vi "ExperimentCode_Serial.vi"() -> ()   [LabVIEW 2017]
uses:
  <vilib>/Analysis/baseanly.llb/Mean (DBL).vi
  <vilib>/Instr/_visa.llb/VISA Configure Serial Port (Instr).vi
  <vilib>/express/express shared/transition.llb/Dynamic To Waveform Array.vi
  <vilib>/express/express signal manip/GetorSetDDTAttributes/Set DDT Attributes/SetT0.vi
  <vilib>/express/express shared/transition.llb/Waveform Array To Dynamic.vi
  <vilib>/express/express signal manip/GetorSetDDTAttributes/Set DDT Attributes/Set DDT Properties.xnode
  <vilib>/Analysis/NI_AALBase.lvlib
panel:
  in  "Tab Control":enum32{"Setup ", "Experiment Controls", "Debug"}(tab)=enum."Experiment Controls"
  in  "Max Torque":dbl=21.3
  in  "Servo 1 Zero Offset":dbl=-9.0
  in  "Servo 2 Zero Offset":dbl=10.0
  in  "Servo 3 Zero Offset":dbl=-9.0
  in  "Servo 4 Zero Offset":dbl
  in  "Servo 5 Zero Offset":dbl
  in  "Servo 5 Torque Intercept":dbl
  in  "Servo 5 Torque Slope":dbl=1.0
  in  "Servo 5 Position Intercept":dbl
  in  "Servo 5 Position Slope":dbl=1.0
  in  "Servo 4 Torque Intercept":dbl=-72.1928
  in  "Servo 4 Torque Slope":dbl=0.002332
  in  "Servo 4 Position Intercept":dbl=97.9723
  in  "Servo 4 Position Slope":dbl=-0.00488
  in  "Servo 3 Torque Intercept":dbl
  in  "Servo 3 Torque Slope":dbl=1.0
  in  "Servo 3 Position Intercept":dbl
  in  "Servo 3 Position Slope":dbl=1.0
  in  "Servo 2 Torque Intercept":dbl
  in  "Servo 2 Torque Slope":dbl=1.0
  in  "Servo 2 Position Intercept":dbl
  in  "Servo 2 Position Slope":dbl=1.0
  in  "Servo 1 Torque Intercept":dbl
  in  "Servo 1 Torque Slope":dbl=1.0
  in  "Servo 1 Position Intercept":dbl
  in  "Servo 1 Position Slope":dbl=1.0
  in  "Plot Last x Seconds":dbl=100.0
  in  "COM Port":refnum<visa-resource-name>
  in  "Buad Rate":i32(ring)=115200 items=["2400"=2400, "4800"=4800, "9600"=9600, "14400"=14400, "19200"=19200, "28800"=28800, "38400"=38400, "57600"=57600, "115200"=115200]
  in  "Lowest Servo Angle":dbl=-65.0
  in  "Highest Servo Angle":dbl=65.0
  in  "Number of Servos":dbl=3.0
  out "Maximum Torque Exceeded":bool
  in  "Amplitude (deg)":dbl=3.0
  in  "Save":bool
  in  "Stop VI":bool
  in  "Sample Frequency":dbl=100.0 step=50.0
  out "Servo Torque":cluster{" Time Offset":dbl, dbl, dbl[][]}(graph)
  in  "Amplitude (cm)":dbl=2.0
  in  "Length of Segments":dbl=10.0
  in  "Number of Waves":dbl=1.0
  in  "Wave Exponential":dbl=2.0
  in  "Frequency":dbl=1.0
  in  "Wave Form":u16(ring) items=["Sine", "Exponentional Sine", "Second Mode Bending", "Flat Plate"]
  in  "Wind Up Waveform":bool
  in  "Mode 1 Amplitude":dbl=0.1 step=0.1
  in  "Mode 2 Amplitude":dbl=0.2 step=0.1
  in  "Mode 1 Phase":dbl step=0.1
  in  "Mode 2 Phase":dbl=0.8499 step=0.1
  in  "Wind Down Waveform":bool
  in  "Wind Down Time":i32=5
  out "Waveform":cluster{"X Nodes":dbl[], "Y Nodes":dbl[]}[](graph)
  in  "Servo Input":bool
  in  "Send To Waveform to MBE":bool
  in  "Servo 5 Input":dbl
  in  "Servo 4 Input":dbl
  in  "Servo 3 Input":dbl
  in  "Servo 2 Input":dbl
  in  "Servo 1  Input":dbl
  out "Minimum or Maximum Angle Exceeded":bool
  in  "Filename":path=path "test.tdms"
  in  "Comment":string
  out "Calculated Sample Frequency":dbl
  out "Specified Time Delay":dbl
  out "Calculated Time Delay":dbl
  out "Time Elapsed":dbl
  out "Output Angles":dbl[](array[numeric])
  out "Input Angles":dbl[](array[numeric])
  out "Pos5 number":dbl
  out "Pos4 number":dbl
  out "Pos3 number":dbl
  out "Pos2 number":dbl
  out "Pos1 number":dbl
  out "Torq1 number":dbl
  out "Torq2 number":dbl
  out "Torq3 number":dbl
  out "Torq4 number":dbl
  out "Torq5 number":dbl
  out "Servo 1 Position":cluster{" Time Offset":dbl, "mean":dbl, dbl[][]}(graph)
  out "Servo 2 Position":cluster{" Time Offset":dbl, "mean":dbl, dbl[][]}(graph)
  out "Servo 3 Position":cluster{" Time Offset":dbl, "mean":dbl, dbl[][]}(graph)
  out "Servo 4 Position":cluster{" Time Offset":dbl, "mean":dbl, dbl[][]}(graph)
  out "Servo 5 Position":cluster{" Time Offset":dbl, "mean":dbl, dbl[][]}(graph)
  out "Sent to Arduino":string
  out "Bytes at port":cluster{i32, dbl, dbl[]}(graph)
  out "Read Buffer":string
  # "deg"
  # "deg"
  # "deg"
  # "deg"
  # "deg"
  # "Waveform"
  # "Manual"
  # "cm"
  # "Hz"
  # "Off"
  # "On"
  # "rad"
  # "rad"
  # "Off"
  # "On"
  # "Hz"
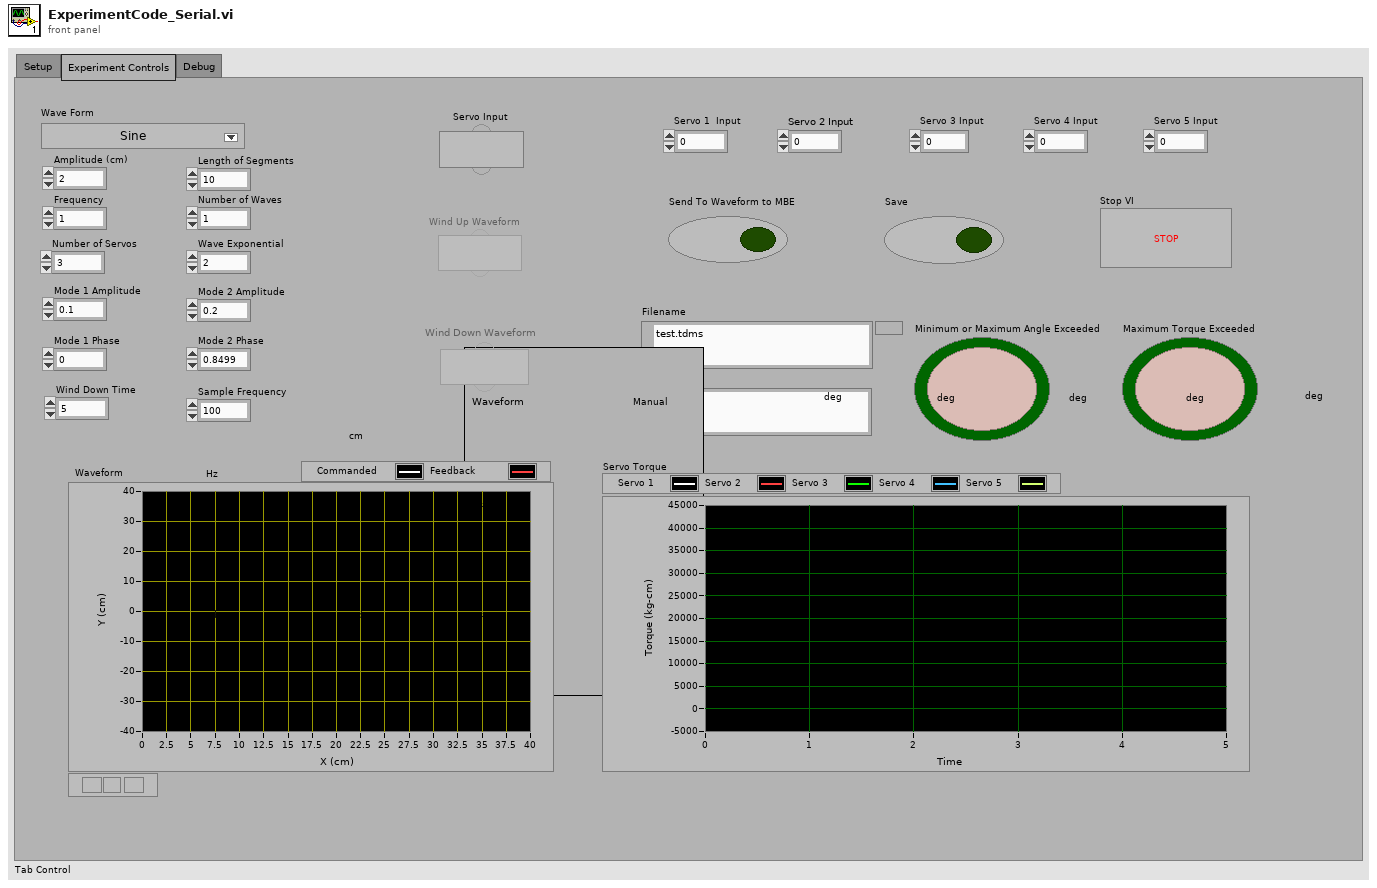
[diagram p1: front panel]
types:
  T1 = enum8{"Enabled", "Disabled", "Disabled and Grayed Out"}
  T2 = cluster{"Amplitude (deg)":dbl, "Amplitude (cm)":dbl, "Frequency":dbl, "Number of Waves":dbl, "Length of Segments":dbl, "Wave Exponential":dbl, "Number of Servos":dbl, "Mode 1 Amplitude":dbl, "Mode 2 Amplitude":dbl, "Mode 1 Phase":dbl, "Mode 2 Phase":dbl}
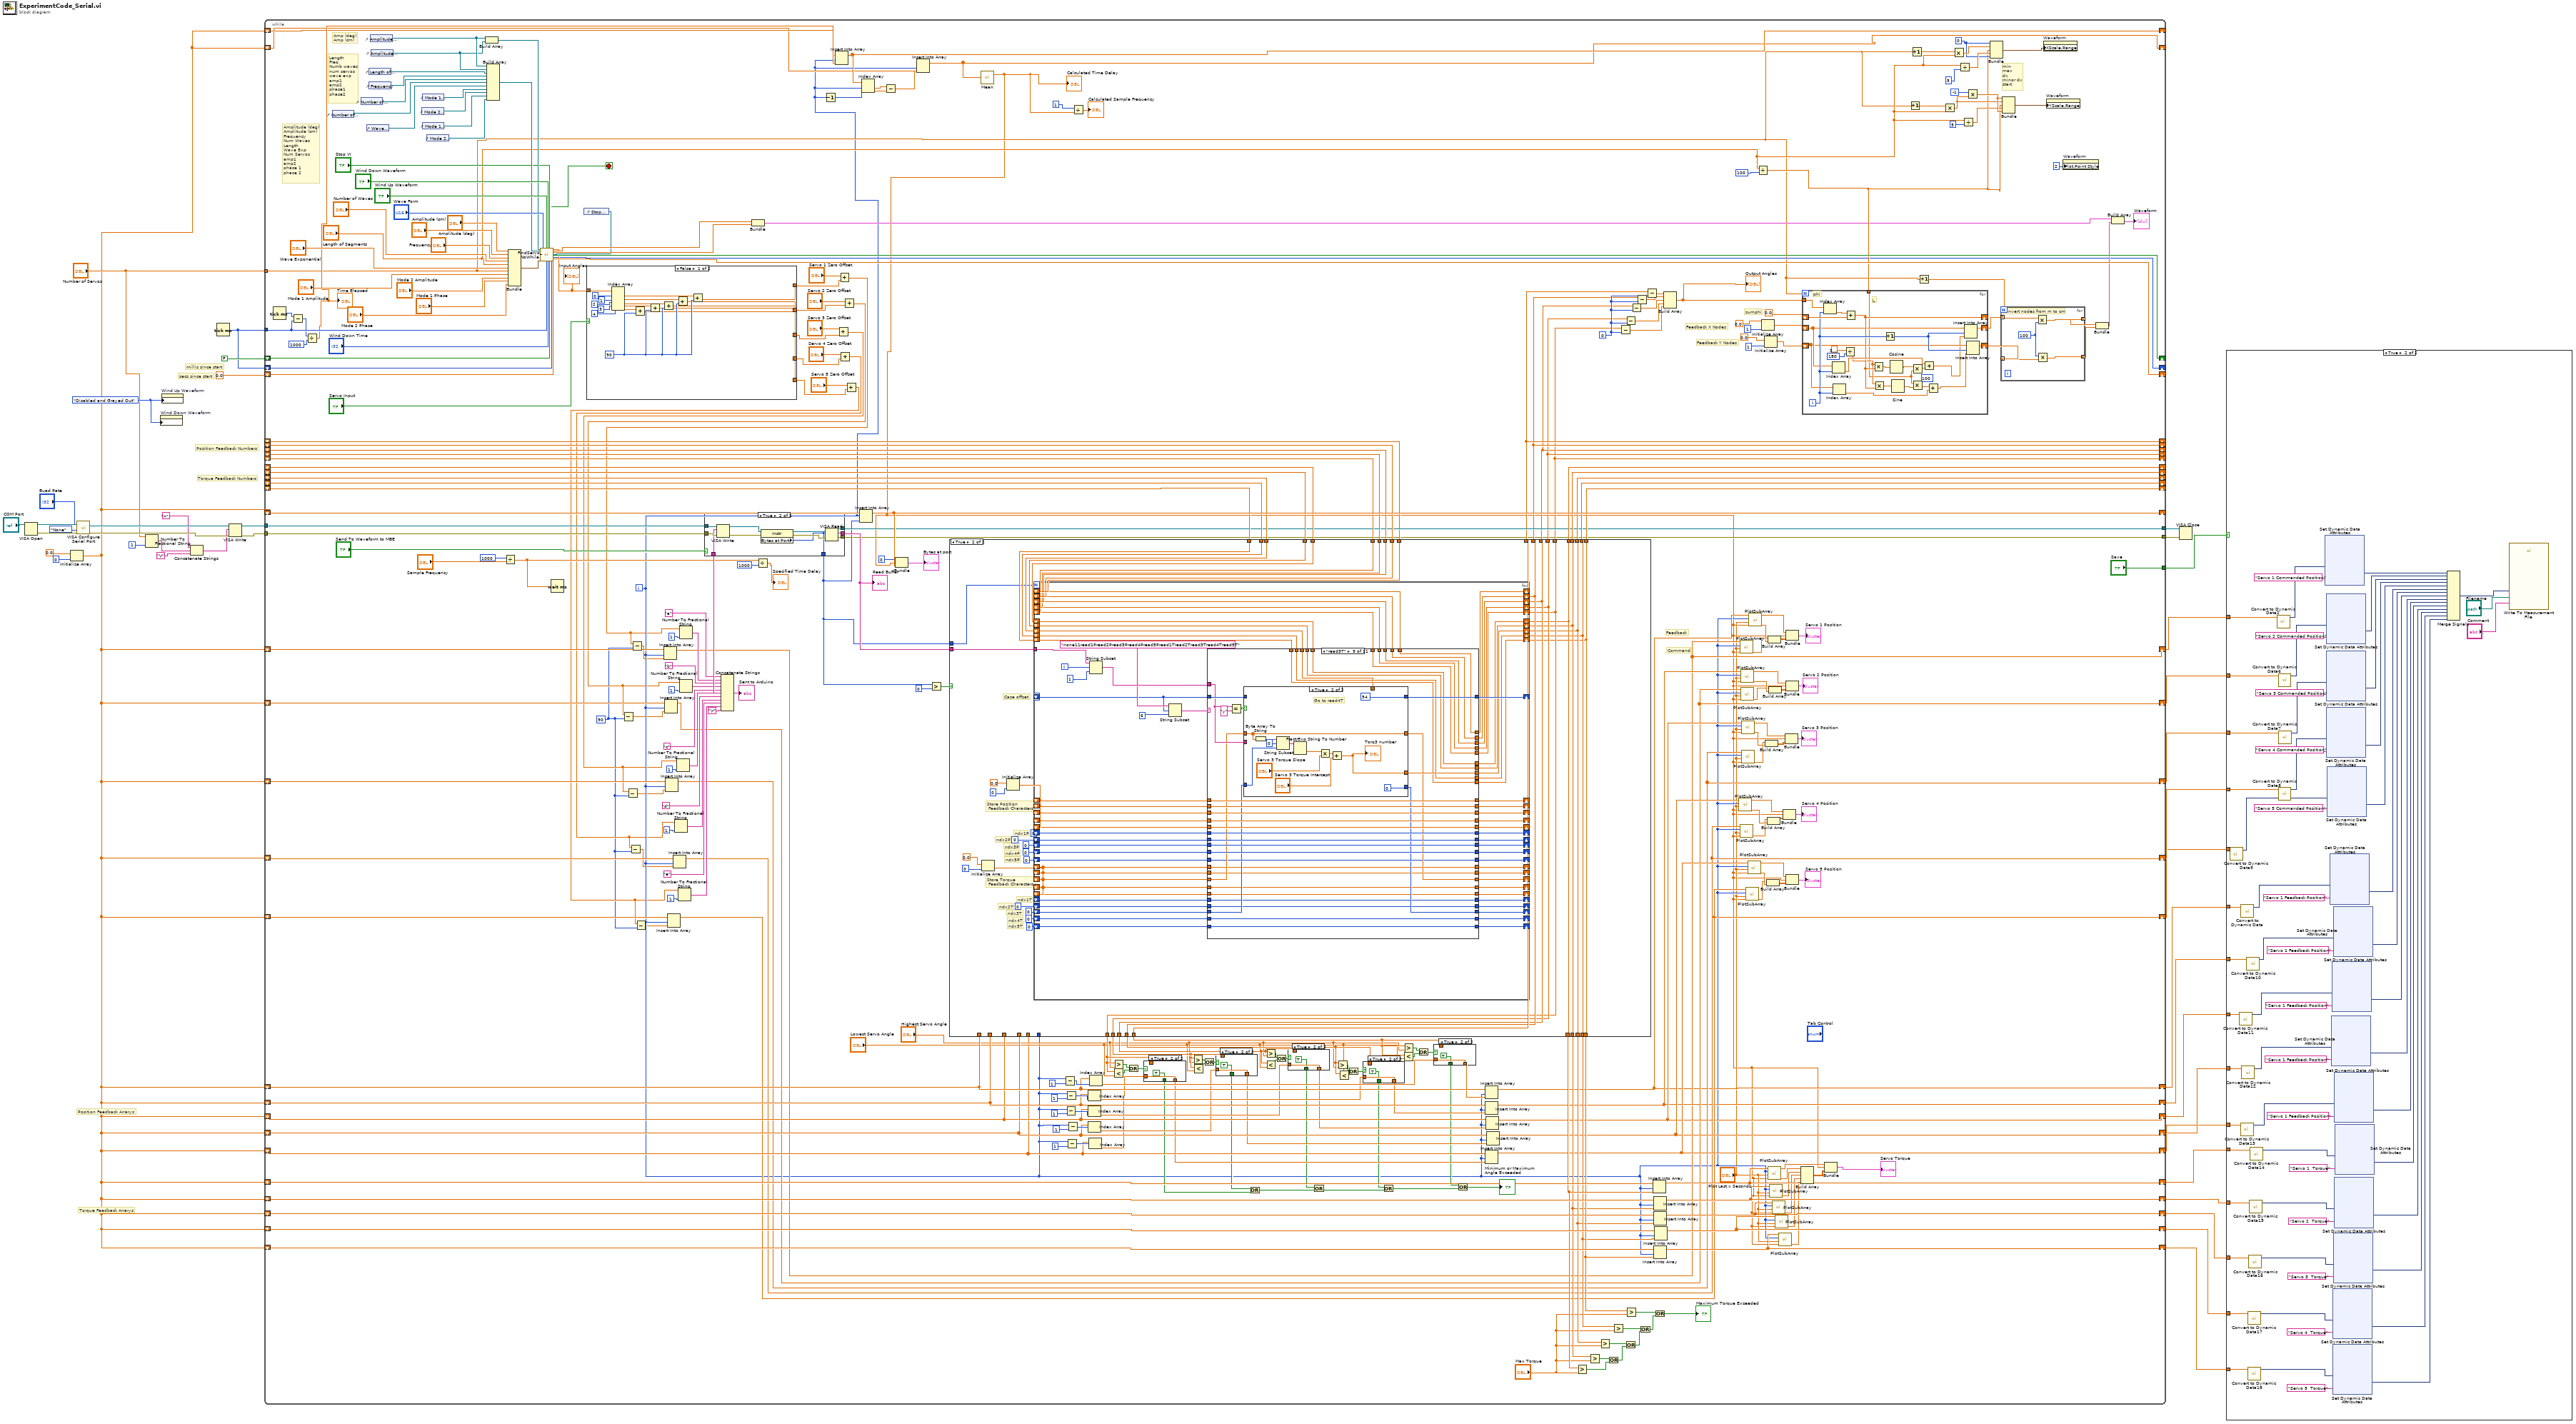
[diagram p0: block diagram]
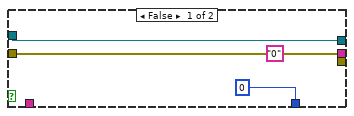
[diagram p3: hidden frame]
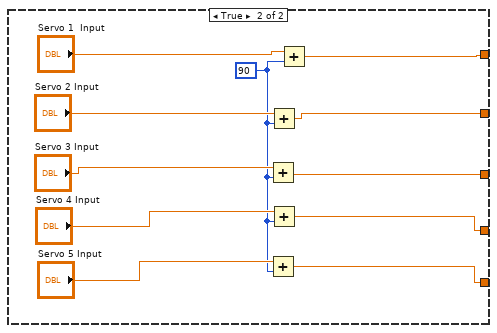
[diagram p4: hidden frame]
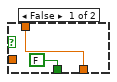
[diagram p5: hidden frame]
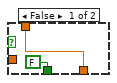
[diagram p6: hidden frame]
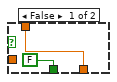
[diagram p7: hidden frame]
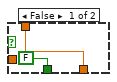
[diagram p8: hidden frame]
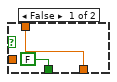
[diagram p9: hidden frame]
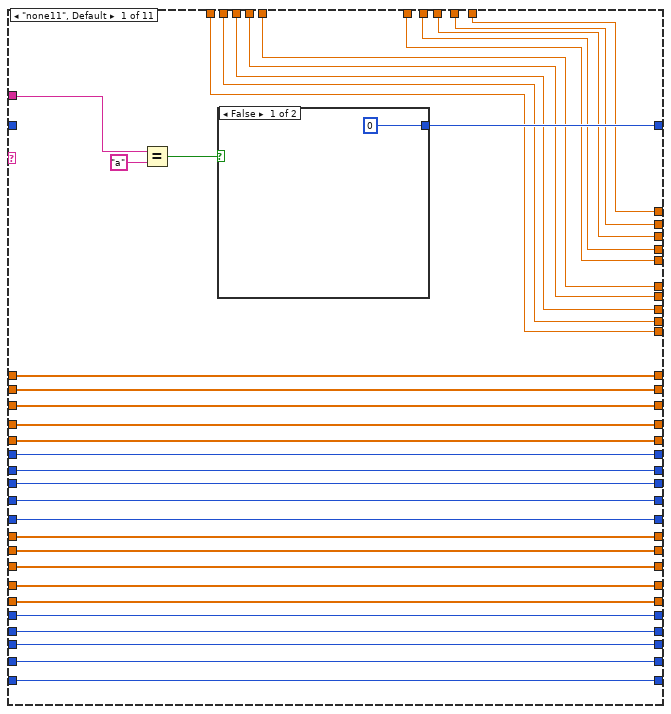
[diagram p11: hidden frame]
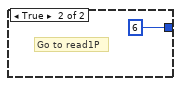
[diagram p12: hidden frame]
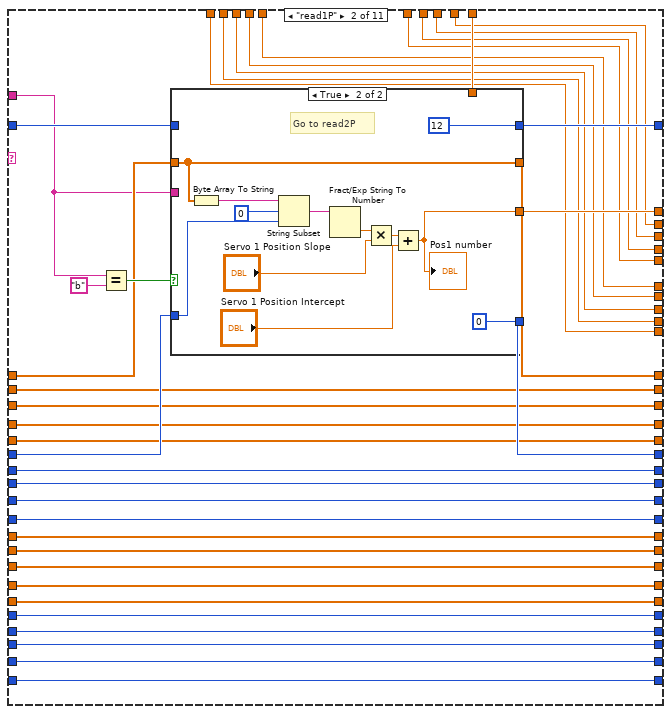
[diagram p13: hidden frame]
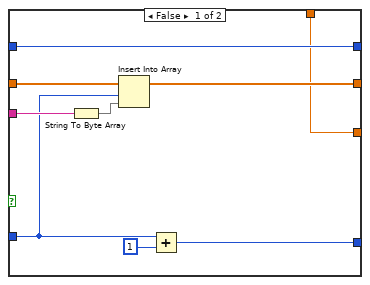
[diagram p14: hidden frame]
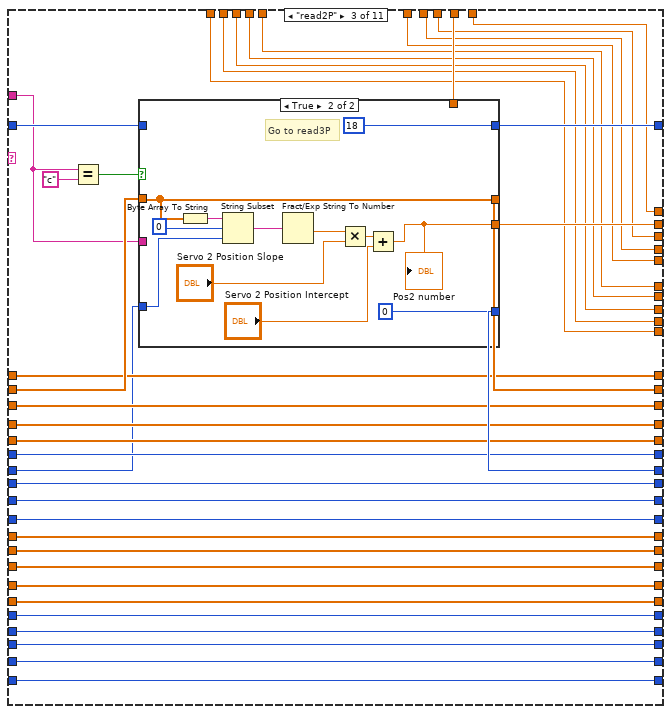
[diagram p15: hidden frame]
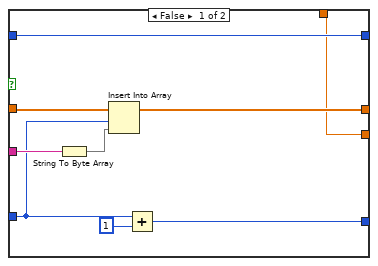
[diagram p16: hidden frame]
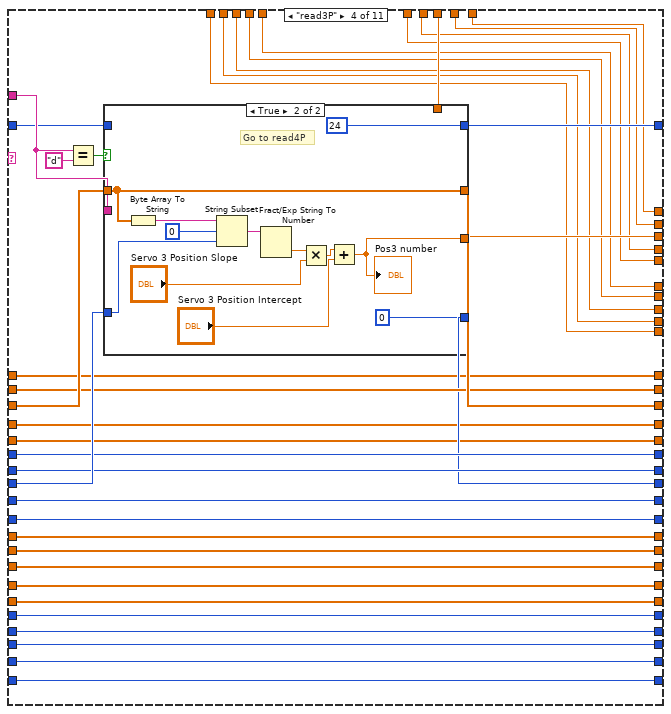
[diagram p17: hidden frame]
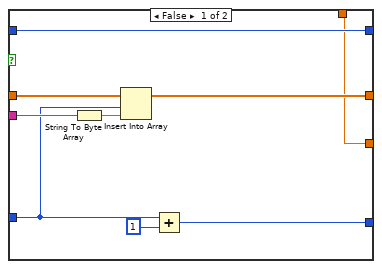
[diagram p18: hidden frame]
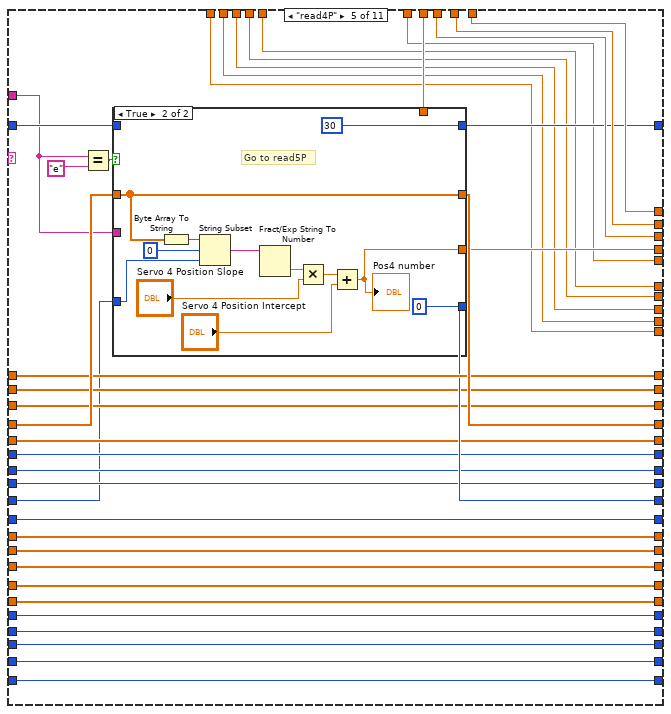
[diagram p19: hidden frame]
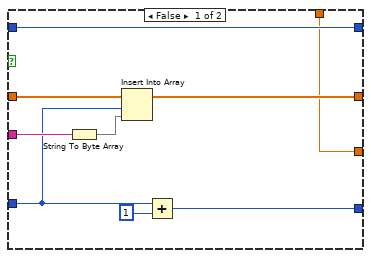
[diagram p20: hidden frame]
diagram:
  w26 = T1."Disabled and Grayed Out" ("Disabled")
  # "secs since start"
  # "millis since start"
  # "Torque Feedback Numbers"
  # "Position Feedback Numbers"
  # "Torque Feedback Arrarys"
  # "Position Feedback Arrarys"
  n1 = VISA Open(VISA resource name="COM Port") -> (VISA resource name=w37:refnum<visa-resource-name>, error out=w35:errorcluster)  [unwired: 4 in]
  n2 = Initialize Array(0.0 ("element"), 0 ("dimension size")) -> (w2:dbl[])
  n3 = call-poly "VISA Configure Serial Port"("VISA resource name"=w37, "baud rate (9600)"="Buad Rate", "parity (0:none)"=enum16{"None", "Odd", "Even", "Mark", "Space"}."None", "error in (no error)"=w35) -> ("VISA resource name out"=w12:refnum<visa-resource-name>, "error out"=w11:errorcluster)  [unwired: 10 in]
  n4 = Number To Fractional String(number="Number of Servos", precision (6)=1) -> (F-format string=w7:string)  [unwired: 2 in]
  n5 = property on="Wind Down Waveform" class="Bool (strict)"("DisabledEnum"=w26) -> ()  [unwired: 2 in, 2 out]
  n6 = property on="Wind Up Waveform" class="Bool (strict)"("DisabledEnum"=w26) -> ()  [unwired: 2 in, 2 out]
  n7 = Concatenate Strings("n", w7, "\r") -> (w3:string)
  n8 = Tick Count (ms)() -> (millisecond timer value=w32:u32)
  n9 = VISA Write(VISA resource name=w12, write buffer=w3, error in (no error)=w11) -> (VISA resource name out=w10:refnum<visa-resource-name>, error out=w9:errorcluster)  [unwired: 1 out]
  n10 = while {
    shift-right: [w343] -> _
    shift-left: w2 -> [w344]
    shift-right: [w70] -> w1
    shift-left: w2 -> [w320]
    shift-right: [w72] -> w25
    shift-left: w2 -> [w319]
    shift-right: [w76] -> w24
    shift-left: w2 -> [w318]
    shift-right: [w78] -> w23
    shift-left: w2 -> [w317]
    shift-right: [w86] -> w22
    shift-left: w2 -> [w316]
    shift-right: [w69] -> w27
    shift-left: w2 -> [w284]
    shift-right: [w71] -> w21
    shift-left: w2 -> [w276]
    shift-right: [w75] -> w20
    shift-left: w2 -> [w273]
    shift-right: [w79] -> w19
    shift-left: w2 -> [w270]
    shift-right: [w85] -> w18
    shift-left: w2 -> [w240]
    shift-right: [w139] -> _
    shift-left: _ -> [w287]
    shift-right: [w138] -> _
    shift-left: _ -> [w306]
    shift-right: [w135] -> _
    shift-left: _ -> [w309]
    shift-right: [w137] -> _
    shift-left: _ -> [w308]
    shift-right: [w136] -> _
    shift-left: _ -> [w307]
    shift-right: [w300] -> _
    shift-left: _ -> [w301]
    shift-right: [w299] -> _
    shift-left: _ -> [w302]
    shift-right: [w298] -> _
    shift-left: _ -> [w303]
    shift-right: [w297] -> _
    shift-left: _ -> [w304]
    shift-right: [w296] -> _
    shift-left: _ -> [w305]
    shift-right: [w180] -> w17
    shift-left: w2 -> [w295]
    shift-right: [w178] -> w16
    shift-left: w2 -> [w294]
    shift-right: [w177] -> w15
    shift-left: w2 -> [w293]
    shift-right: [w176] -> w14
    shift-left: w2 -> [w292]
    shift-right: [w179] -> w13
    shift-left: w2 -> [w291]
    tunnel: w9 -> [w239]
    tunnel: w32 -> [w103]
    shift-right: [w233] -> _
    shift-left: FALSE -> [w228]
    shift-right: [w93] -> _
    shift-left: w32 -> [w99]
    shift-right: [w232] -> _
    shift-left: 0.0 ("S since stop Shift Out") -> [w100]
    tunnel: ["Save"] -> w30
    tunnel: w10 -> [w238]
    tunnel: [w288] -> w29
    tunnel: [w108] -> w28
    shift-right: [w90] -> _
    shift-left: w2 -> [w97]
    tunnel: "Number of Servos" -> [w92]
    shift-right: [w87] -> _
    shift-left: w2 -> [w88]
    i -> [w67]
    stop <- w190 stop-if-true
    w44 = 90
    w124 = 0
    w140 = 0
    # "min\nmax\ndx\nminor dx\nstart"
    # "Feedback Y Nodes"
    # "Feedback X Nodes"
    # "sumphi"
    # "Command"
    # "Feedback"
    # "Amplitude (deg)\nAmplitude (cm)\nFrequency\nNum Waves\nLength\nWave Exp\nNum Servos\namp1\namp2\nphase 1\nphase 2"
    # "Amp (deg)\nAmp (cm)"
    # "Length\nFreq\nNumb waves\nnum servos\nwave exp\namp1\namp2\nphase1\nphase2"
    n11 = Tick Count (ms)() -> (millisecond timer value=w104:u32)
    n12 = Subtract(x=w104, y=w103) -> (x-y=w102:u32)
    n13 = Divide(x=w102, y=1000) -> (x/y=w98:dbl)
    "Time Elapsed" <- w98
    n14 = control-ref of="Number of Servos"() -> (w91:refnum<vi>)
    n15 = control-ref of="Number of Waves"() -> (w213:refnum<vi>)
    n16 = control-ref of="Wave Exponential"() -> (w212:refnum<vi>)
    n17 = control-ref of="Length of Segments"() -> (w215:refnum<vi>)
    n18 = control-ref of="Frequency"() -> (w214:refnum<vi>)
    n19 = control-ref of="Amplitude (deg)"() -> (w195:refnum<vi>)
    n20 = control-ref of="Amplitude (cm)"() -> (w194:refnum<vi>)
    n21 = control-ref of="Mode 2 Amplitude"() -> (w210:refnum<vi>)
    n22 = control-ref of="Mode 1 Amplitude"() -> (w211:refnum<vi>)
    n23 = control-ref of="Mode 1 Phase"() -> (w209:refnum<vi>)
    n24 = control-ref of="Mode 2 Phase"() -> (w208:refnum<vi>)
    n25 = Build Array(w195, w194) -> (w197:refnum<vi>[])
    n26 = Build Array(w195, w194, w215, w214, w213, w91, w212, w211, w210, w209, w208) -> (w196:refnum<vi>[])
    n27 = Divide(x=1000, y="Sample Frequency") -> (x/y=w106:dbl)
    n28 = Bundle("Amplitude (deg)"="Amplitude (deg)", "Amplitude (cm)"="Amplitude (cm)", "Frequency"="Frequency", "Number of Waves"="Number of Waves", "Length of Segments"="Length of Segments", "Wave Exponential"="Wave Exponential", "Number of Servos"=w92, "Mode 1 Amplitude"="Mode 1 Amplitude", "Mode 2 Amplitude"="Mode 2 Amplitude", "Mode 1 Phase"="Mode 1 Phase", "Mode 2 Phase"="Mode 2 Phase") -> (w198:T2)  [unwired: 1 in]
    n29 = Wait (ms)(milliseconds to wait=w106) -> ()  [unwired: 1 out]
    n30 = control-ref of="Stop Reference"() -> (w227:refnum<vi>)
    n31 = call "FindServo_NoWhile.vi"("Amplitude Reference Array"=w197, "Parameter Reference Arrary"=w196, "Parameter Cluster"=w198, "Wave Form"="Wave Form", "Wind Up"="Wind Up Waveform", "Start Time (Tick Count-millis)"=w103, "Wind Down"="Wind Down Waveform", "Wind Down Time"="Wind Down Time", "Stop In"="Stop VI", "Stop Pressed Shift In (False)"=w228, "Ms Since Stop Shift In (Start Time)"=w99, "Stop In Reference"=w227, "S since stop Shift In"=w100) -> ("Stop Out"=w190:bool, "phi"=w109:dbl[], "X Nodes"=w231:dbl[], "Y Nodes"=w230:dbl[], "Stop Pressed Shift Out (False)"=w233:bool, "MS Since Stop Shift Out"=w93:u32, "S since stop Shift Out"=w232:dbl)  [unwired: 8 in]
    "Input Angles" <- w109
    n32 = case shown="False" "Servo Input" {
      tunnel: [w393 w416] -> w221
      tunnel: [w392 w408] -> w220
      tunnel: [w391 w407] -> w219
      tunnel: [w390 w412] -> w218
      tunnel: [w389 w413] -> w217
      tunnel: w109 -> [w405 _]
      frame False {
        w394 = 90
        n33 = Index Array(array=w405, index #1=0, index #2=1, index #3=2, index #4=3, index #5=4) -> (element #1=w399:dbl, element #2=w398:dbl, element #3=w397:dbl, element #4=w396:dbl, element #5=w395:dbl)
        n34 = Add(x=w395, y=w394) -> (x+y=w389:dbl)
        n35 = Add(x=w396, y=w394) -> (x+y=w390:dbl)
        n36 = Add(x=w397, y=w394) -> (x+y=w391:dbl)
        n37 = Add(x=w398, y=w394) -> (x+y=w392:dbl)
        n38 = Add(x=w399, y=w394) -> (x+y=w393:dbl)
      }
      frame True {
        w406 = 90
        n39 = Add(x="Servo 3 Input", y=w406) -> (x+y=w407:dbl)
        n40 = Add(x="Servo 5 Input", y=w406) -> (x+y=w413:dbl)
        n41 = Add(x="Servo 2 Input", y=w406) -> (x+y=w408:dbl)
        n42 = Add(x="Servo 4 Input", y=w406) -> (x+y=w412:dbl)
        n43 = Add(x="Servo 1  Input", y=w406) -> (x+y=w416:dbl)
      }
    }
    n44 = Bundle("X Nodes"=w231, "Y Nodes"=w230) -> (w119:cluster{"X Nodes":dbl[], "Y Nodes":dbl[]})  [unwired: 1 in]
    n45 = Divide(x=w106, y=1000) -> (x/y=→"Specified Time Delay":dbl)
    n46 = Decrement(x=w67) -> (x-1=w94:i32)
    n47 = Insert Into Array(array=w97, index=w67, new element=w98) -> (w90:dbl[])
    n48 = Add(x="Servo 3 Zero Offset", y=w219) -> (x+y=w49:dbl)
    n49 = Subtract(x=w49, y=w44) -> (x-y=w50:dbl)
    n50 = Insert Into Array(array=w318, index=w67, new element=w50) -> (w76:dbl[])
    n51 = Number To Fractional String(number=w49, precision (6)=1) -> (F-format string=w339:string)  [unwired: 2 in]
    n52 = Add(x="Servo 1 Zero Offset", y=w221) -> (x+y=w53:dbl)
    n53 = Subtract(x=w53, y=w44) -> (x-y=w54:dbl)
    n54 = Insert Into Array(array=w320, index=w67, new element=w54) -> (w70:dbl[])
    n55 = Number To Fractional String(number=w53, precision (6)=1) -> (F-format string=w341:string)  [unwired: 2 in]
    n56 = Add(x="Servo 4 Zero Offset", y=w218) -> (x+y=w47:dbl)
    n57 = Subtract(x=w47, y=w44) -> (x-y=w48:dbl)
    n58 = Insert Into Array(array=w317, index=w67, new element=w48) -> (w78:dbl[])
    n59 = Number To Fractional String(number=w47, precision (6)=1) -> (F-format string=w332:string)  [unwired: 2 in]
    n60 = Add(x="Servo 2 Zero Offset", y=w220) -> (x+y=w51:dbl)
    n61 = Subtract(x=w51, y=w44) -> (x-y=w52:dbl)
    n62 = Insert Into Array(array=w319, index=w67, new element=w52) -> (w72:dbl[])
    n63 = Number To Fractional String(number=w51, precision (6)=1) -> (F-format string=w340:string)  [unwired: 2 in]
    n64 = Add(x="Servo 5 Zero Offset", y=w217) -> (x+y=w45:dbl)
    n65 = Subtract(x=w45, y=w44) -> (x-y=w46:dbl)
    n66 = Insert Into Array(array=w316, index=w67, new element=w46) -> (w86:dbl[])
    n67 = Number To Fractional String(number=w45, precision (6)=1) -> (F-format string=w331:string)  [unwired: 2 in]
    n68 = Concatenate Strings("a", w341, "b", w340, "c", w339, "d", w332, "e", w331, "\r") -> (w342:string)
    "Sent to Arduino" <- w342
    n69 = case shown="True" "Send To Waveform to MBE" {
      tunnel: w342 -> [_ w378]
      tunnel: ["0" w388] -> w327
      tunnel: [w376 w387] -> w108
      tunnel: [w377 w386] -> w288
      tunnel: [0 w381] -> w193
      tunnel: w239 -> [w376 w380]
      tunnel: w238 -> [w377 w379]
      frame False {
      }
      frame True {
        n70 = VISA Write(VISA resource name=w379, write buffer=w378, error in (no error)=w380) -> (VISA resource name out=w385:refnum<visa-resource-name>, error out=w382:errorcluster)  [unwired: 1 out]
        n71 = property class="Instr"(reference=w385, error in=w382) -> (reference out=w384:refnum<visa-resource-name>, error out=w383:errorcluster, "Bytes at Port"=w381:u32)
        n72 = VISA Read(VISA resource name=w384, byte count=w381, error in (no error)=w383) -> (VISA resource name out=w386:refnum<visa-resource-name>, read buffer=w388:string, error out=w387:errorcluster)  [unwired: 1 out]
      }
    }
    "Read Buffer" <- w327
    n73 = Insert Into Array(array=w344, index=w67, new element=w193) -> (w343:dbl[])
    n74 = Index Array(array=w90, index #1=w67, index #2=w94) -> (element #1=w96:dbl, element #2=w95:dbl)
    n75 = Subtract(x=w96, y=w95) -> (x-y=w89:dbl)
    n76 = Insert Into Array(array=w88, index=w67, new element=w89) -> (w87:dbl[])
    n77 = Greater?(x=w193, y=0) -> (0:w290:bool)
    n78 = case shown="True" w290 {
      tunnel: w193 -> [_ w447]
      tunnel: w327 -> [_ w485]
      tunnel: [w446 w459] -> w279
      tunnel: w67 -> [_ _]
      tunnel: w284 -> [_ _]
      tunnel: [w445 w458] -> w261
      tunnel: [w444 w457] -> w255
      tunnel: [w443 w456] -> w249
      tunnel: [w442 w455] -> w245
      tunnel: w276 -> [_ _]
      tunnel: w273 -> [_ _]
      tunnel: w270 -> [_ _]
      tunnel: w240 -> [_ _]
      tunnel: w287 -> [w446 w476]
      tunnel: w306 -> [w445 w475]
      tunnel: w309 -> [w444 w474]
      tunnel: w308 -> [w443 w473]
      tunnel: w307 -> [w442 w472]
      tunnel: [w446 w459] -> w139
      tunnel: [w445 w458] -> w138
      tunnel: [w444 w457] -> w135
      tunnel: [w443 w456] -> w137
      tunnel: [w442 w455] -> w136
      tunnel: w305 -> [w437 w449]
      tunnel: w304 -> [w438 w451]
      tunnel: w303 -> [w439 w471]
      tunnel: w302 -> [w440 w470]
      tunnel: w301 -> [w441 w469]
      tunnel: [w441 w454] -> w300
      tunnel: [w440 w453] -> w299
      tunnel: [w439 w452] -> w298
      tunnel: [w438 w450] -> w297
      tunnel: [w437 w448] -> w296
      tunnel: [w441 w454] -> w168
      tunnel: [w440 w453] -> w164
      tunnel: [w439 w452] -> w165
      tunnel: [w438 w450] -> w166
      tunnel: [w437 w448] -> w167
      frame False {
      }
      frame True {
        # "Store Torque\n Feedback Characters"
        # "ndx5T"
        # "ndx4T"
        # "ndx3T"
        # "ndx2T"
        # "ndx1T"
        # "Store Position\n Feedback Characters"
        # "ndx5P"
        # "ndx4P"
        # "ndx3P"
        # "ndx2P"
        # "ndx1P"
        # "Case offset"
        n79 = Initialize Array(0.0 ("element"), 0 ("dimension size")) -> (w466:dbl[])
        n80 = Initialize Array(0.0 ("element"), 0 ("dimension size")) -> (w479:dbl[])
        n81 = for {
          N: w447 -> [_]
          tunnel: w485 -> [w553]
          shift-right: [w551] -> _
          shift-left: 1 -> [w496]
          shift-right: [w550] -> _
          shift-left: 0 -> [w549]
          shift-right: [w547] -> _
          shift-left: w479 -> [w548]
          shift-right: [w545] -> _
          shift-left: w479 -> [w546]
          shift-right: [w541] -> _
          shift-left: 0 -> [w544]
          shift-right: [w542] -> _
          shift-left: 0 -> [w543]
          shift-right: [w539] -> _
          shift-left: w479 -> [w540]
          shift-right: [w531] -> _
          shift-left: w479 -> [w538]
          shift-right: [w532] -> _
          shift-left: w479 -> [w537]
          shift-right: [w535] -> _
          shift-left: 0 -> [w536]
          shift-right: [w533] -> _
          shift-left: 0 -> [w534]
          shift-right: [w518] -> _
          shift-left: w466 -> [w519]
          shift-right: [w517] -> _
          shift-left: w466 -> [w516]
          shift-right: [w515] -> _
          shift-left: w466 -> [w514]
          shift-right: [w513] -> _
          shift-left: w466 -> [w512]
          shift-right: [w511] -> _
          shift-left: w466 -> [w510]
          shift-right: [w509] -> _
          shift-left: 0 -> [w508]
          shift-right: [w507] -> _
          shift-left: 0 -> [w506]
          shift-right: [w505] -> _
          shift-left: 0 -> [w504]
          shift-right: [w502] -> _
          shift-left: 0 -> [w503]
          shift-right: [w501] -> _
          shift-left: 0 -> [w500]
          shift-right: [w495] -> w459
          shift-left: w476 -> [w526]
          shift-right: [w494] -> w458
          shift-left: w475 -> [w530]
          shift-right: [w493] -> w457
          shift-left: w474 -> [w529]
          shift-right: [w492] -> w456
          shift-left: w473 -> [w528]
          shift-right: [w491] -> w455
          shift-left: w472 -> [w527]
          shift-right: [w490] -> w454
          shift-left: w469 -> [w520]
          shift-right: [w489] -> w453
          shift-left: w470 -> [w521]
          shift-right: [w488] -> w452
          shift-left: w471 -> [w522]
          shift-right: [w487] -> w450
          shift-left: w451 -> [w523]
          shift-right: [w486] -> w448
          shift-left: w449 -> [w524]
          i -> [w497]
          n82 = String Subset(string=w553, offset (0)=w497, length (rest)=1 ("length (rest)")) -> (substring=w525:string)
          n83 = String Subset(string="none11read1Pread2Pread3Pread4Pread5Pread1Tread2Tread3Tread4Tread5T", offset (0)=w496, length (rest)=6 ("length (rest)")) -> (substring=w499:string)
          n84 = case shown="\"read3T\"" w499 {
            tunnel: w525 -> [w588 w622 w678 w732 w799 w858 w919 w978 w1037 w1096 w1155]
            tunnel: [w585 w625 w680 w739 w785 w861 w922 w981 w1040 w1099 w1158] -> w551
            tunnel: [w584 w620 w682 w744 w797 w851 w914 w973 w1032 w1091 w1150] -> w550
            tunnel: w549 -> [w584 w621 w682 w744 w797 w851 w914 w973 w1032 w1091 w1150]
            tunnel: w548 -> [w581 w623 w677 w727 w803 w855 w918 w977 w1036 w1095 w1154]
            tunnel: [w581 w626 w677 w727 w803 w855 w918 w977 w1036 w1095 w1154] -> w547
            tunnel: w546 -> [w582 w619 w687 w740 w795 w854 w917 w976 w1035 w1094 w1153]
            tunnel: [w582 w619 w686 w740 w795 w854 w917 w976 w1035 w1094 w1153] -> w545
            tunnel: w544 -> [w583 w615 w665 w743 w796 w850 w913 w972 w1031 w1090 w1149]
            tunnel: [w583 w615 w685 w743 w796 w850 w913 w972 w1031 w1090 w1149] -> w541
            tunnel: w496 -> [_ w624 w681 w724 w800 w860 w921 w980 w1039 w1098 w1157]
            tunnel: w543 -> [w578 w614 w679 w745 w792 w849 w912 w971 w1030 w1089 w1148]
            tunnel: [w578 w614 w679 w736 w792 w849 w912 w971 w1030 w1089 w1148] -> w542
            tunnel: w540 -> [w575 w618 w676 w742 w794 w853 w916 w975 w1034 w1093 w1152]
            tunnel: [w575 w618 w676 w741 w794 w853 w916 w975 w1034 w1093 w1152] -> w539
            tunnel: w538 -> [w576 w617 w675 w735 w805 w852 w915 w974 w1033 w1092 w1151]
            tunnel: w537 -> [w577 w616 w674 w734 w793 w863 w906 w965 w1017 w1076 w1135]
            tunnel: w536 -> [w580 w613 w673 w738 w784 w848 w911 w970 w1029 w1088 w1147]
            tunnel: [w580 w613 w673 w738 w798 w848 w911 w970 w1029 w1088 w1147] -> w535
            tunnel: w534 -> [w579 w612 w672 w737 w791 w857 w903 w954 w1014 w1070 w1132]
            tunnel: [w579 w612 w672 w737 w791 w856 w903 w954 w1014 w1070 w1132] -> w533
            tunnel: [w577 w616 w674 w734 w793 w862 w906 w965 w1017 w1076 w1135] -> w532
            tunnel: [w576 w617 w675 w735 w804 w852 w915 w974 w1033 w1092 w1151] -> w531
            tunnel: [w570 w611 w669 w725 w786 w847 w910 w969 w1028 w1087 w1146] -> w495
            tunnel: w526 -> [w570 w610 w669 w725 w786 w847 w910 w969 w1028 w1087 w1146]
            tunnel: [w574 w609 w671 w731 w790 w842 w907 w966 w1025 w1084 w1143] -> w494
            tunnel: w530 -> [w574 w609 w670 w731 w790 w842 w907 w966 w1025 w1084 w1143]
            tunnel: [w573 w608 w666 w730 w787 w845 w909 w968 w1027 w1086 w1145] -> w493
            tunnel: w529 -> [w573 w608 w666 w729 w787 w845 w909 w968 w1027 w1086 w1145]
            tunnel: [w572 w607 w668 w728 w789 w843 w908 w967 w1026 w1085 w1144] -> w492
            tunnel: w528 -> [w572 w607 w668 w728 w788 w843 w908 w967 w1026 w1085 w1144]
            tunnel: [w571 w606 w667 w726 w768 w846 w899 w949 w1023 w1083 w1142] -> w491
            tunnel: w527 -> [w571 w606 w667 w726 w768 w844 w899 w949 w1023 w1083 w1142]
            tunnel: w524 -> [w565 w601 w660 w719 w779 w837 w887 w945 w1018 w1077 w1141]
            tunnel: w523 -> [w566 w602 w661 w720 w780 w838 w888 w946 w1020 w1082 w1136]
            tunnel: w522 -> [w567 w603 w662 w721 w781 w839 w889 w947 w1024 w1079 w1137]
            tunnel: w521 -> [w568 w604 w663 w722 w782 w840 w890 w951 w1021 w1080 w1138]
            tunnel: w520 -> [w569 w605 w664 w723 w783 w841 w900 w950 w1022 w1081 w1139]
            tunnel: [w569 w605 w664 w723 w783 w841 w898 w950 w1022 w1081 w1139] -> w490
            tunnel: [w568 w604 w663 w722 w782 w840 w890 w948 w1021 w1080 w1138] -> w489
            tunnel: [w567 w603 w662 w721 w781 w839 w889 w947 w1019 w1079 w1137] -> w488
            tunnel: [w566 w602 w661 w720 w780 w838 w888 w946 w1020 w1078 w1136] -> w487
            tunnel: [w565 w601 w660 w719 w779 w837 w887 w945 w1018 w1077 w1140] -> w486
            tunnel: w519 -> [w564 w600 w659 w718 w778 w836 w905 w962 w1011 w1073 w1122]
            tunnel: [w564 w600 w659 w718 w778 w836 w904 w962 w1011 w1073 w1122] -> w518
            tunnel: [w563 w599 w658 w717 w777 w835 w897 w963 w1010 w1072 w1123] -> w517
            tunnel: w516 -> [w563 w599 w658 w717 w777 w835 w897 w964 w1010 w1072 w1123]
            tunnel: [w562 w598 w657 w716 w776 w834 w896 w961 w1015 w1071 w1124] -> w515
            tunnel: w514 -> [w562 w598 w657 w716 w776 w834 w896 w961 w1016 w1071 w1124]
            tunnel: [w561 w597 w656 w715 w775 w833 w895 w960 w1009 w1075 w1125] -> w513
            tunnel: w512 -> [w561 w597 w656 w715 w775 w833 w895 w960 w1009 w1074 w1125]
            tunnel: [w560 w596 w655 w714 w774 w832 w894 w959 w1008 w1066 w1134] -> w511
            tunnel: w510 -> [w560 w596 w655 w714 w774 w832 w894 w959 w1008 w1066 w1133]
            tunnel: [w559 w595 w654 w713 w773 w831 w901 w958 w1007 w1067 w1126] -> w509
            tunnel: w508 -> [w559 w595 w654 w713 w773 w831 w902 w958 w1007 w1067 w1126]
            tunnel: [w558 w594 w653 w712 w772 w830 w893 w953 w1006 w1065 w1127] -> w507
            tunnel: w506 -> [w558 w594 w653 w712 w772 w830 w893 w952 w1006 w1065 w1127]
            tunnel: [w557 w593 w652 w711 w771 w829 w892 w957 w1013 w1064 w1128] -> w505
            tunnel: w504 -> [w557 w593 w652 w711 w771 w829 w892 w957 w1012 w1064 w1128]
            tunnel: w503 -> [w556 w592 w651 w710 w770 w828 w891 w956 w1005 w1068 w1129]
            tunnel: [w556 w592 w651 w710 w770 w828 w891 w956 w1005 w1069 w1129] -> w502
            tunnel: [w555 w591 w650 w709 w769 w827 w886 w955 w1004 w1063 w1131] -> w501
            tunnel: w500 -> [w555 w591 w650 w709 w769 w827 w886 w955 w1004 w1063 w1130]
            frame "none11", Default {
              n85 = Equal?(x=w588, y="a") -> (x = y?=w586:bool)
              n86 = case shown="False" w586 {
                tunnel: [0 6] -> w585
                frame False {
                }
                frame True {
                  # "Go to read1P"
                }
              }
            }
            frame "read1P" {
              n87 = Equal?(x=w622, y="b") -> (x = y?=w627:bool)
              n88 = case shown="True" w627 {
                tunnel: [w637 0] -> w620
                tunnel: w623 -> [w631 w645]
                tunnel: [w635 w645] -> w626
                tunnel: w622 -> [w634 _]
                tunnel: [w632 12] -> w625
                tunnel: w624 -> [w632 _]
                tunnel: w621 -> [w630 w644]
                tunnel: [w629 w642] -> w611
                tunnel: w610 -> [w629 _]
                frame False {
                  n89 = String To Byte Array(string=w634) -> (unsigned byte array=w633:u8[])
                  n90 = Insert Into Array(array=w631, index=w630, new element=w633) -> (w635:dbl[])
                  n91 = Add(x=w630, y=1) -> (x+y=w637:i32)
                }
                frame True {
                  # "Go to read2P"
                  n92 = Byte Array To String(unsigned byte array=w645) -> (string=w646:string)
                  n93 = String Subset(string=w646, offset (0)=0, length (rest)=w644) -> (substring=w643:string)
                  n94 = Fract/Exp String To Number(string=w643) -> (number=w641:dbl)  [unwired: 3 in, 1 out]
                  n95 = Multiply(x=w641, y="Servo 1 Position Slope") -> (x*y=w640:dbl)
                  n96 = Add(x=w640, y="Servo 1 Position Intercept") -> (x+y=w642:dbl)
                  "Pos1 number" <- w642
                }
              }
            }
            frame "read2P" {
              n97 = Equal?(x=w678, y="c") -> (x = y?=w683:bool)
              n98 = case shown="True" w683 {
                tunnel: [w696 0] -> w685
                tunnel: w665 -> [w690 w705]
                tunnel: w687 -> [w694 w703]
                tunnel: [w693 w703] -> w686
                tunnel: w678 -> [w692 _]
                tunnel: [w689 18] -> w680
                tunnel: w681 -> [w689 _]
                tunnel: [w688 w699] -> w671
                tunnel: w670 -> [w688 _]
                frame False {
                  n99 = String To Byte Array(string=w692) -> (unsigned byte array=w691:u8[])
                  n100 = Insert Into Array(array=w694, index=w690, new element=w691) -> (w693:dbl[])
                  n101 = Add(x=w690, y=1) -> (x+y=w696:i32)
                }
                frame True {
                  # "Go to read3P"
                  n102 = Byte Array To String(unsigned byte array=w703) -> (string=w702:string)
                  n103 = String Subset(string=w702, offset (0)=0, length (rest)=w705) -> (substring=w704:string)
                  n104 = Fract/Exp String To Number(string=w704) -> (number=w700:dbl)  [unwired: 3 in, 1 out]
                  n105 = Multiply(x=w700, y="Servo 2 Position Slope") -> (x*y=w701:dbl)
                  n106 = Add(x=w701, y="Servo 2 Position Intercept") -> (x+y=w699:dbl)
                  "Pos2 number" <- w699
                }
              }
            }
            frame "read3P" {
              n107 = Equal?(x=w732, y="d") -> (x = y?=w746:bool)
              n108 = case shown="True" w746 {
                tunnel: [w755 0] -> w736
                tunnel: w745 -> [w749 w762]
                tunnel: w742 -> [w753 w763]
                tunnel: [w752 w763] -> w741
                tunnel: w732 -> [w751 _]
                tunnel: [w748 24] -> w739
                tunnel: w724 -> [w748 _]
                tunnel: [w747 w756] -> w730
                tunnel: w729 -> [w747 _]
                frame False {
                  n109 = String To Byte Array(string=w751) -> (unsigned byte array=w750:u8[])
                  n110 = Insert Into Array(array=w753, index=w749, new element=w750) -> (w752:dbl[])
                  n111 = Add(x=w749, y=1) -> (x+y=w755:i32)
                }
                frame True {
                  # "Go to read4P"
                  n112 = Byte Array To String(unsigned byte array=w763) -> (string=w764:string)
                  n113 = String Subset(string=w764, offset (0)=0, length (rest)=w762) -> (substring=w761:string)
                  n114 = Fract/Exp String To Number(string=w761) -> (number=w759:dbl)  [unwired: 3 in, 1 out]
                  n115 = Multiply(x=w759, y="Servo 3 Position Slope") -> (x*y=w760:dbl)
                  n116 = Add(x=w760, y="Servo 3 Position Intercept") -> (x+y=w756:dbl)
                  "Pos3 number" <- w756
                }
              }
            }
            frame "read4P" {
              n117 = Equal?(x=w799, y="e") -> (x = y?=w801:bool)
              n118 = case shown="True" w801 {
                tunnel: [w814 0] -> w798
                tunnel: w784 -> [w808 w822]
                tunnel: w805 -> [w812 w823]
                tunnel: [w811 w823] -> w804
                tunnel: w799 -> [w810 _]
                tunnel: [w807 30] -> w785
                tunnel: w800 -> [w807 _]
                tunnel: [w806 w819] -> w789
                tunnel: w788 -> [w806 _]
                frame False {
                  n119 = String To Byte Array(string=w810) -> (unsigned byte array=w809:u8[])
                  n120 = Insert Into Array(array=w812, index=w808, new element=w809) -> (w811:dbl[])
                  n121 = Add(x=w808, y=1) -> (x+y=w814:i32)
                }
                frame True {
                  # "Go to read5P"
                  n122 = Byte Array To String(unsigned byte array=w823) -> (string=w824:string)
                  n123 = String Subset(string=w824, offset (0)=0, length (rest)=w822) -> (substring=w821:string)
                  n124 = Fract/Exp String To Number(string=w821) -> (number=w818:dbl)  [unwired: 3 in, 1 out]
                  n125 = Multiply(x=w818, y="Servo 4 Position Slope") -> (x*y=w820:dbl)
                  n126 = Add(x=w820, y="Servo 4 Position Intercept") -> (x+y=w819:dbl)
                  "Pos4 number" <- w819
                }
              }
            }
            frame "read5P" {
              n127 = Equal?(x=w858, y="v") -> (x = y?=w859:bool)
              n128 = case shown="True" w859 {
                tunnel: [w873 0] -> w856
                tunnel: w857 -> [w867 w880]
                tunnel: w863 -> [w871 w881]
                tunnel: [w870 w881] -> w862
                tunnel: w858 -> [w869 _]
                tunnel: [w866 36] -> w861
                tunnel: w860 -> [w866 _]
                tunnel: [w865 w875] -> w846
                tunnel: w844 -> [w865 _]
                frame False {
                  n129 = String To Byte Array(string=w869) -> (unsigned byte array=w868:u8[])
                  n130 = Insert Into Array(array=w871, index=w867, new element=w868) -> (w870:dbl[])
                  n131 = Add(x=w867, y=1) -> (x+y=w873:i32)
                }
                frame True {
                  # "Go to read1T"
                  n132 = Byte Array To String(unsigned byte array=w881) -> (string=w882:string)
                  n133 = String Subset(string=w882, offset (0)=0, length (rest)=w880) -> (substring=w879:string)
                  n134 = Fract/Exp String To Number(string=w879) -> (number=w877:dbl)  [unwired: 3 in, 1 out]
                  n135 = Multiply(x=w877, y="Servo 5 Position Slope") -> (x*y=w878:dbl)
                  n136 = Add(x=w878, y="Servo 5 Position Intercept") -> (x+y=w875:dbl)
                  "Pos5 number" <- w875
                }
              }
            }
            frame "read1T" {
              n137 = Equal?(x=w919, y="w") -> (x = y?=w920:bool)
              n138 = case shown="True" w920 {
                tunnel: [w932 0] -> w901
                tunnel: w902 -> [w926 w938]
                tunnel: w905 -> [w930 w940]
                tunnel: [w929 w940] -> w904
                tunnel: w919 -> [w928 _]
                tunnel: [w925 42] -> w922
                tunnel: w921 -> [w925 _]
                tunnel: [w924 w935] -> w898
                tunnel: w900 -> [w924 _]
                frame False {
                  n139 = String To Byte Array(string=w928) -> (unsigned byte array=w927:u8[])
                  n140 = Insert Into Array(array=w930, index=w926, new element=w927) -> (w929:dbl[])
                  n141 = Add(x=w926, y=1) -> (x+y=w932:i32)
                }
                frame True {
                  # "Go to read2T"
                  n142 = Byte Array To String(unsigned byte array=w940) -> (string=w941:string)
                  n143 = String Subset(string=w941, offset (0)=0, length (rest)=w938) -> (substring=w939:string)
                  n144 = Fract/Exp String To Number(string=w939) -> (number=w936:dbl)  [unwired: 3 in, 1 out]
                  n145 = Multiply(x=w936, y="Servo 1 Torque Slope") -> (x*y=w937:dbl)
                  n146 = Add(x=w937, y="Servo 1 Torque Intercept") -> (x+y=w935:dbl)
                  "Torq1 number" <- w935
                }
              }
            }
            frame "read2T" {
              n147 = Equal?(x=w978, y="x") -> (x = y?=w979:bool)
              n148 = case shown="True" w979 {
                tunnel: [w991 0] -> w953
                tunnel: w952 -> [w985 w997]
                tunnel: w964 -> [w989 w999]
                tunnel: [w988 w999] -> w963
                tunnel: w978 -> [w987 _]
                tunnel: [w984 48] -> w981
                tunnel: w980 -> [w984 _]
                tunnel: [w983 w994] -> w948
                tunnel: w951 -> [w983 _]
                frame False {
                  n149 = String To Byte Array(string=w987) -> (unsigned byte array=w986:u8[])
                  n150 = Insert Into Array(array=w989, index=w985, new element=w986) -> (w988:dbl[])
                  n151 = Add(x=w985, y=1) -> (x+y=w991:i32)
                }
                frame True {
                  # "Go to read3T"
                  n152 = Byte Array To String(unsigned byte array=w999) -> (string=w1000:string)
                  n153 = String Subset(string=w1000, offset (0)=0, length (rest)=w997) -> (substring=w998:string)
                  n154 = Fract/Exp String To Number(string=w998) -> (number=w995:dbl)  [unwired: 3 in, 1 out]
                  n155 = Multiply(x=w995, y="Servo 2 Torque Slope") -> (x*y=w996:dbl)
                  n156 = Add(x=w996, y="Servo 2 Torque Intercept") -> (x+y=w994:dbl)
                  "Torq2 number" <- w994
                }
              }
            }
            frame "read3T" {
              n157 = Equal?(x=w1037, y="y") -> (x = y?=w1038:bool)
              n158 = case shown="True" w1038 {
                tunnel: [w1050 0] -> w1013
                tunnel: w1012 -> [w1044 w1056]
                tunnel: w1016 -> [w1048 w1058]
                tunnel: [w1047 w1058] -> w1015
                tunnel: w1037 -> [w1046 _]
                tunnel: [w1043 54] -> w1040
                tunnel: w1039 -> [w1043 _]
                tunnel: [w1042 w1054] -> w1019
                tunnel: w1024 -> [w1042 _]
                frame False {
                  n159 = String To Byte Array(string=w1046) -> (unsigned byte array=w1045:u8[])
                  n160 = Insert Into Array(array=w1048, index=w1044, new element=w1045) -> (w1047:dbl[])
                  n161 = Add(x=w1044, y=1) -> (x+y=w1050:i32)
                }
                frame True {
                  # "Go to read4T"
                  n162 = Byte Array To String(unsigned byte array=w1058) -> (string=w1059:string)
                  n163 = String Subset(string=w1059, offset (0)=0, length (rest)=w1056) -> (substring=w1057:string)
                  n164 = Fract/Exp String To Number(string=w1057) -> (number=w1053:dbl)  [unwired: 3 in, 1 out]
                  n165 = Multiply(x=w1053, y="Servo 3 Torque Slope") -> (x*y=w1055:dbl)
                  n166 = Add(x=w1055, y="Servo 3 Torque Intercept") -> (x+y=w1054:dbl)
                  "Torq3 number" <- w1054
                }
              }
            }
            frame "read4T" {
              n167 = Equal?(x=w1096, y="z") -> (x = y?=w1097:bool)
              n168 = case shown="True" w1097 {
                tunnel: [w1109 0] -> w1069
                tunnel: w1068 -> [w1103 w1115]
                tunnel: w1074 -> [w1107 w1117]
                tunnel: [w1106 w1117] -> w1075
                tunnel: w1096 -> [w1105 _]
                tunnel: [w1102 60] -> w1099
                tunnel: w1098 -> [w1102 _]
                tunnel: [w1101 w1112] -> w1078
                tunnel: w1082 -> [w1101 _]
                frame False {
                  n169 = String To Byte Array(string=w1105) -> (unsigned byte array=w1104:u8[])
                  n170 = Insert Into Array(array=w1107, index=w1103, new element=w1104) -> (w1106:dbl[])
                  n171 = Add(x=w1103, y=1) -> (x+y=w1109:i32)
                }
                frame True {
                  # "Go to read5T"
                  n172 = Byte Array To String(unsigned byte array=w1117) -> (string=w1118:string)
                  n173 = String Subset(string=w1118, offset (0)=0, length (rest)=w1115) -> (substring=w1116:string)
                  n174 = Fract/Exp String To Number(string=w1116) -> (number=w1113:dbl)  [unwired: 3 in, 1 out]
                  n175 = Multiply(x=w1113, y="Servo 4 Torque Slope") -> (x*y=w1114:dbl)
                  n176 = Add(x=w1114, y="Servo 4 Torque Intercept") -> (x+y=w1112:dbl)
                  "Torq4 number" <- w1112
                }
              }
            }
            frame "read5T" {
              n177 = Equal?(x=w1155, y="!") -> (x = y?=w1156:bool)
              n178 = case shown="True" w1156 {
                tunnel: [w1168 0] -> w1131
                tunnel: w1130 -> [w1162 w1174]
                tunnel: w1133 -> [w1166 w1176]
                tunnel: [w1165 w1176] -> w1134
                tunnel: w1155 -> [w1164 _]
                tunnel: [w1161 0] -> w1158
                tunnel: w1157 -> [w1161 _]
                tunnel: [w1160 w1169] -> w1140
                tunnel: w1141 -> [w1160 _]
                frame False {
                  n179 = String To Byte Array(string=w1164) -> (unsigned byte array=w1163:u8[])
                  n180 = Insert Into Array(array=w1166, index=w1162, new element=w1163) -> (w1165:dbl[])
                  n181 = Add(x=w1162, y=1) -> (x+y=w1168:i32)
                }
                frame True {
                  # "Go to none11"
                  n182 = Byte Array To String(unsigned byte array=w1176) -> (string=w1177:string)
                  n183 = String Subset(string=w1177, offset (0)=0, length (rest)=w1174) -> (substring=w1175:string)
                  n184 = Fract/Exp String To Number(string=w1175) -> (number=w1172:dbl)  [unwired: 3 in, 1 out]
                  n185 = Multiply(x=w1172, y="Servo 5 Torque Slope") -> (x*y=w1173:dbl)
                  n186 = Add(x=w1173, y="Servo 5 Torque Intercept") -> (x+y=w1169:dbl)
                  "Torq5 number" <- w1169
                }
              }
            }
          }
        }
      }
    }
    n187 = call-poly <vilib>:"Mean.vi"("X"=w87) -> ("mean"=w42:dbl)  [unwired: 1 out]
    "Calculated Time Delay" <- w42
    n188 = Bundle(0, "mean"=w42, w343) -> (→"Bytes at port":cluster{i32, "mean":dbl, dbl[]})  [unwired: 1 in]
    n189 = Subtract(x=w67, y=1) -> (x-y=w286:i32)
    n190 = Subtract(x=w67, y=1) -> (x-y=w275:i32)
    n191 = Subtract(x=w67, y=1) -> (x-y=w278:i32)
    n192 = Subtract(x=w67, y=1) -> (x-y=w269:i32)
    n193 = Subtract(x=w67, y=1) -> (x-y=w272:i32)
    n194 = Divide(x=1, y=w42) -> (x/y=→"Calculated Sample Frequency":dbl)
    n195 = Index Array(array=w273, index=w275) -> (element=w257:dbl)
    n196 = Index Array(array=w276, index=w278) -> (element=w262:dbl)
    n197 = Index Array(array=w270, index=w272) -> (element=w251:dbl)
    n198 = Index Array(array=w240, index=w269) -> (element=w242:dbl)
    n199 = Index Array(array=w284, index=w286) -> (element=w281:dbl)
    n200 = Less?(x=w245, y="Lowest Servo Angle") -> (x < y?=w246:bool)
    n201 = Greater?(x=w245, y="Highest Servo Angle") -> (0:w248:bool)
    n202 = Or(x=w248, y=w246) -> (x .or. y?=w247:bool)
    n203 = case shown="True" w247 {
      tunnel: w242 -> [_ w420]
      tunnel: w245 -> [w418 _]
      tunnel: [w418 w420] -> w241
      tunnel: [FALSE TRUE] -> w188
      frame False {
      }
      frame True {
      }
    }
    n204 = Greater?(x=w249, y="Highest Servo Angle") -> (0:w252:bool)
    n205 = Less?(x=w249, y="Lowest Servo Angle") -> (x < y?=w253:bool)
    n206 = Or(x=w252, y=w253) -> (x .or. y?=w254:bool)
    n207 = case shown="True" w254 {
      tunnel: w251 -> [_ w424]
      tunnel: w249 -> [w422 _]
      tunnel: [w422 w424] -> w250
      tunnel: [FALSE TRUE] -> w189
      frame False {
      }
      frame True {
      }
    }
    n208 = Or(x=w189, y=w188) -> (x .or. y?=w186:bool)
    n209 = Greater?(x=w255, y="Highest Servo Angle") -> (0:w260:bool)
    n210 = Less?(x=w255, y="Lowest Servo Angle") -> (x < y?=w258:bool)
    n211 = Or(x=w260, y=w258) -> (x .or. y?=w259:bool)
    n212 = case shown="True" w259 {
      tunnel: w257 -> [_ w428]
      tunnel: w255 -> [w426 _]
      tunnel: [w426 w428] -> w256
      tunnel: [FALSE TRUE] -> w187
      frame False {
      }
      frame True {
      }
    }
    n213 = Or(x=w187, y=w186) -> (x .or. y?=w184:bool)
    n214 = Greater?(x=w261, y="Highest Servo Angle") -> (0:w266:bool)
    n215 = Less?(x=w261, y="Lowest Servo Angle") -> (x < y?=w264:bool)
    n216 = Or(x=w266, y=w264) -> (x .or. y?=w265:bool)
    n217 = case shown="True" w265 {
      tunnel: w262 -> [_ w432]
      tunnel: w261 -> [w430 _]
      tunnel: [w430 w432] -> w263
      tunnel: [FALSE TRUE] -> w185
      frame False {
      }
      frame True {
      }
    }
    n218 = Or(x=w185, y=w184) -> (x .or. y?=w182:bool)
    n219 = Less?(x=w279, y="Lowest Servo Angle") -> (x < y?=w280:bool)
    n220 = Greater?(x=w279, y="Highest Servo Angle") -> (0:w283:bool)
    n221 = Or(x=w283, y=w280) -> (x .or. y?=w282:bool)
    n222 = case shown="True" w282 {
      tunnel: w281 -> [_ w436]
      tunnel: w279 -> [w434 _]
      tunnel: [w434 w436] -> w267
      tunnel: [FALSE TRUE] -> w183
      frame False {
      }
      frame True {
      }
    }
    n223 = Or(x=w183, y=w182) -> (x .or. y?=→"Minimum or Maximum Angle Exceeded":bool)
    n224 = Insert Into Array(array=w284, index=w67, new element=w267) -> (w69:dbl[])
    n225 = Insert Into Array(array=w276, index=w67, new element=w263) -> (w71:dbl[])
    n226 = Insert Into Array(array=w240, index=w67, new element=w241) -> (w85:dbl[])
    n227 = Insert Into Array(array=w273, index=w67, new element=w256) -> (w75:dbl[])
    n228 = Insert Into Array(array=w270, index=w67, new element=w250) -> (w79:dbl[])
    n229 = Greater?(x=w168, y="Max Torque") -> (0:w162:bool)
    n230 = Greater?(x=w164, y="Max Torque") -> (0:w161:bool)
    n231 = Greater?(x=w165, y="Max Torque") -> (0:w160:bool)
    n232 = Or(x=w161, y=w162) -> (x .or. y?=w159:bool)
    n233 = Greater?(x=w166, y="Max Torque") -> (0:w158:bool)
    n234 = Subtract(x=w136, y=w140) -> (x-y=w141:dbl)
    n235 = Subtract(x=w137, y=w140) -> (x-y=w142:dbl)
    n236 = Or(x=w160, y=w159) -> (x .or. y?=w155:bool)
    n237 = Greater?(x=w167, y="Max Torque") -> (0:w157:bool)
    n238 = Subtract(x=w135, y=w140) -> (x-y=w143:dbl)
    n239 = Subtract(x=w138, y=w140) -> (x-y=w144:dbl)
    n240 = Or(x=w158, y=w155) -> (x .or. y?=w156:bool)
    n241 = Subtract(x=w139, y=w140) -> (x-y=w145:dbl)
    n242 = Insert Into Array(array=w295, index=w67, new element=w168) -> (w180:dbl[])
    n243 = Insert Into Array(array=w294, index=w67, new element=w164) -> (w178:dbl[])
    n244 = Insert Into Array(array=w291, index=w67, new element=w167) -> (w179:dbl[])
    n245 = Or(x=w157, y=w156) -> (x .or. y?=→"Maximum Torque Exceeded":bool)
    n246 = Insert Into Array(array=w293, index=w67, new element=w165) -> (w177:dbl[])
    n247 = Insert Into Array(array=w292, index=w67, new element=w166) -> (w176:dbl[])
    n248 = Build Array(w145, w144, w143, w142, w141) -> (w110:dbl[])
    "Output Angles" <- w110
    n249 = call "PlotSubArray.vi"("Time Step (s)"=w42, "Plot Last x Seconds"="Plot Last x Seconds", "Iteration"=w67, "Array"=w79) -> ("Sub Array"=w60:dbl[], "Time Offset"=w77:dbl)  [unwired: 6 in]
    n250 = call "PlotSubArray.vi"("Time Step (s)"=w42, "Plot Last x Seconds"="Plot Last x Seconds", "Iteration"=w67, "Array"=w70) -> ("Sub Array"=w66:dbl[])  [unwired: 6 in, 1 out]
    n251 = call "PlotSubArray.vi"("Time Step (s)"=w42, "Plot Last x Seconds"="Plot Last x Seconds", "Iteration"=w67, "Array"=w78) -> ("Sub Array"=w59:dbl[])  [unwired: 6 in, 1 out]
    n252 = call "PlotSubArray.vi"("Time Step (s)"=w42, "Plot Last x Seconds"="Plot Last x Seconds", "Iteration"=w67, "Array"=w71) -> ("Sub Array"=w64:dbl[], "Time Offset"=w73:dbl)  [unwired: 6 in]
    n253 = call "PlotSubArray.vi"("Time Step (s)"=w42, "Plot Last x Seconds"="Plot Last x Seconds", "Iteration"=w67, "Array"=w72) -> ("Sub Array"=w63:dbl[])  [unwired: 6 in, 1 out]
    n254 = call "PlotSubArray.vi"("Time Step (s)"=w42, "Plot Last x Seconds"="Plot Last x Seconds", "Iteration"=w67, "Array"=w76) -> ("Sub Array"=w62:dbl[])  [unwired: 6 in, 1 out]
    n255 = call "PlotSubArray.vi"("Time Step (s)"=w42, "Plot Last x Seconds"="Plot Last x Seconds", "Iteration"=w67, "Array"=w75) -> ("Sub Array"=w61:dbl[], "Time Offset"=w74:dbl)  [unwired: 6 in]
    n256 = call "PlotSubArray.vi"("Time Step (s)"=w42, "Plot Last x Seconds"="Plot Last x Seconds", "Iteration"=w67, "Array"=w86) -> ("Sub Array"=w57:dbl[])  [unwired: 6 in, 1 out]
    n257 = call "PlotSubArray.vi"("Time Step (s)"=w42, "Plot Last x Seconds"="Plot Last x Seconds", "Iteration"=w67, "Array"=w85) -> ("Sub Array"=w58:dbl[], "Time Offset"=w84:dbl)  [unwired: 6 in]
    n258 = call "PlotSubArray.vi"("Time Step (s)"=w42, "Plot Last x Seconds"="Plot Last x Seconds", "Iteration"=w67, "Array"=w69) -> ("Sub Array"=w65:dbl[], "Time Offset"=w68:dbl)  [unwired: 6 in]
    n259 = Divide(x="Length of Segments", y=100) -> (x/y=w121:dbl)
    n260 = Initialize Array(0.0 ("element"), 1 ("dimension size")) -> (w148:dbl[])
    n261 = Initialize Array(0.0 ("element"), 1 ("dimension size")) -> (w147:dbl[])
    n262 = Build Array(w62, w61) -> (w310:dbl[][])
    n263 = Build Array(w57, w58) -> (w83:dbl[][])
    n264 = Build Array(w59, w60) -> (w81:dbl[][])
    n265 = Build Array(w66, w65) -> (w312:dbl[][])
    n266 = call "PlotSubArray.vi"("Time Step (s)"=w42, "Plot Last x Seconds"="Plot Last x Seconds", "Iteration"=w67, "Array"=w180) -> ("Sub Array"=w175:dbl[], "Time Offset"=w56:dbl)  [unwired: 6 in]
    n267 = Build Array(w63, w64) -> (w311:dbl[][])
    n268 = call "PlotSubArray.vi"("Time Step (s)"=w42, "Plot Last x Seconds"="Plot Last x Seconds", "Iteration"=w67, "Array"=w178) -> ("Sub Array"=w174:dbl[])  [unwired: 6 in, 1 out]
    n269 = call "PlotSubArray.vi"("Time Step (s)"=w42, "Plot Last x Seconds"="Plot Last x Seconds", "Iteration"=w67, "Array"=w177) -> ("Sub Array"=w173:dbl[])  [unwired: 6 in, 1 out]
    n270 = call "PlotSubArray.vi"("Time Step (s)"=w42, "Plot Last x Seconds"="Plot Last x Seconds", "Iteration"=w67, "Array"=w176) -> ("Sub Array"=w172:dbl[])  [unwired: 6 in, 1 out]
    n271 = call "PlotSubArray.vi"("Time Step (s)"=w42, "Plot Last x Seconds"="Plot Last x Seconds", "Iteration"=w67, "Array"=w179) -> ("Sub Array"=w171:dbl[])  [unwired: 6 in, 1 out]
    n272 = Bundle("Time Offset"=w77, "mean"=w42, w81) -> (→"Servo 4 Position":cluster{" Time Offset":dbl, "mean":dbl, dbl[][]})  [unwired: 1 in]
    n273 = Bundle("Time Offset"=w74, "mean"=w42, w310) -> (→"Servo 3 Position":cluster{" Time Offset":dbl, "mean":dbl, dbl[][]})  [unwired: 1 in]
    n274 = Bundle("Time Offset"=w73, "mean"=w42, w311) -> (→"Servo 2 Position":cluster{" Time Offset":dbl, "mean":dbl, dbl[][]})  [unwired: 1 in]
    n275 = Bundle("Time Offset"=w84, "mean"=w42, w83) -> (→"Servo 5 Position":cluster{" Time Offset":dbl, "mean":dbl, dbl[][]})  [unwired: 1 in]
    n276 = Bundle("Time Offset"=w68, "mean"=w42, w312) -> (→"Servo 1 Position":cluster{" Time Offset":dbl, "mean":dbl, dbl[][]})  [unwired: 1 in]
    n277 = Build Array(w175, w174, w173, w172, w171) -> (w170:dbl[][])
    n278 = for {
      N: w92 -> [_]
      shift-right: [w356] -> _
      shift-left: 0.0 -> [w373]
      tunnel: w110 -> [w372]
      shift-right: [w366] -> w117
      shift-left: w148 -> [w354]
      shift-right: [w365] -> w116
      shift-left: w147 -> [w353]
      tunnel: w121 -> [w352]
      i -> [w364]
      (unwired) 100
      # "phi"
      # "L"
      n279 = Index Array(array=w372, index=w364) -> (element=w371:dbl)
      n280 = Index Array(array=w354, index=w364) -> (element=w370:dbl)
      n281 = Index Array(array=w353, index=w364) -> (element=w367:dbl)
      n282 = Divide(x=3.141592653589793, y=180) -> (x/y=w355:dbl)
      n283 = Add(x=w371, y=w373) -> (x+y=w356:dbl)
      n284 = Multiply(x=w355, y=w356) -> (x*y=w358:dbl)
      n285 = Multiply(x=w355, y=w356) -> (x*y=w357:dbl)
      n286 = Increment(x=w364) -> (x+1=w363:i32)
      n287 = Cosine(x=w358) -> (cos(x)=w362:dbl)
      n288 = Sine(x=w357) -> (sin(x)=w361:dbl)
      n289 = Multiply(x=w362, y=w352) -> (x*y=w369:dbl)
      n290 = Multiply(x=w352, y=w361) -> (x*y=w368:dbl)
      n291 = Add(x=w370, y=w369) -> (x+y=w351:dbl)
      n292 = Add(x=w368, y=w367) -> (x+y=w350:dbl)
      n293 = Insert Into Array(array=w354, index=w363, new element=w351) -> (w366:dbl[])
      n294 = Insert Into Array(array=w353, index=w363, new element=w350) -> (w365:dbl[])
    }
    n295 = Bundle("Time Offset"=w56, "mean"=w42, w170) -> (→"Servo Torque":cluster{" Time Offset":dbl, "mean":dbl, dbl[][]})  [unwired: 1 in]
    n296 = Increment(x=w92) -> (x+1=w134:dbl)
    n297 = Increment(x=w92) -> (x+1=w131:dbl)
    n298 = Increment(x=w92) -> (x+1=w118:dbl)
    n299 = Multiply(x=w134, y="Length of Segments") -> (x*y=w132:dbl)
    n300 = Multiply(x=w131, y="Length of Segments") -> (x*y=w128:dbl)
    n301 = Divide(x="Length of Segments", y=5) -> (x/y=w129:dbl)
    n302 = Divide(x="Length of Segments", y=5) -> (x/y=w130:dbl)
    n303 = Multiply(x=-1, y=w132) -> (x*y=w133:dbl)
    n304 = Bundle(w124, w128, w121, w129, w124) -> (w123:cluster{i32, dbl, dbl, dbl, i32})  [unwired: 1 in]
    n305 = for {
      N: w118 -> [_]
      tunnel: w117 -> [w349] mode=indexing
      tunnel: w116 -> [w347] mode=indexing
      tunnel: [w346] -> w114 mode=indexing
      tunnel: [w345] -> w113 mode=indexing
      w348 = 100
      # "Convert nodes from m to cm"
      n306 = Multiply(x=w349, y=w348) -> (x*y=w346:dbl)
      n307 = Multiply(x=w348, y=w347) -> (x*y=w345:dbl)
    }
    n308 = Bundle(w133, w132, w121, w130, w133) -> (w122:cluster{dbl, dbl, dbl, dbl, dbl})  [unwired: 1 in]
    n309 = property on="Waveform" class="XYGraph (strict)"("XScale.Range"=w123) -> ()  [unwired: 2 in, 2 out]
    n310 = property on="Waveform" class="XYGraph (strict)"("YScale.Range"=w122) -> ()  [unwired: 2 in, 2 out]
    n311 = property on="Waveform" class="XYGraph (strict)"("Plot.Point Style"=u8 2) -> ()  [unwired: 2 in, 2 out]
    n312 = Bundle(w114, w113) -> (w112:cluster{dbl[], dbl[]})  [unwired: 1 in]
    n313 = Build Array(w119, w112) -> (→"Waveform":cluster{"X Nodes":dbl[], "Y Nodes":dbl[]}[])
  }
  n314 = VISA Close(VISA resource name=w29, error in (no error)=w28) -> ()  [unwired: 1 out]
  n315 = case shown="True" w30 {
    tunnel: w1 -> [_ w1243]
    tunnel: w27 -> [_ w1242]
    tunnel: w25 -> [_ w1229]
    tunnel: w24 -> [_ w1228]
    tunnel: w23 -> [_ w1227]
    tunnel: w22 -> [_ w1226]
    tunnel: w21 -> [_ w1217]
    tunnel: w20 -> [_ w1216]
    tunnel: w19 -> [_ w1215]
    tunnel: w18 -> [_ w1214]
    tunnel: w17 -> [_ w1212]
    tunnel: w16 -> [_ w1202]
    tunnel: w15 -> [_ w1201]
    tunnel: w14 -> [_ w1200]
    tunnel: w13 -> [_ w1199]
    frame False {
    }
    frame True {
      n316 = call "Convert to Dynamic Data9"("Array"=w1226) -> ("Dynamic Data Type"=w1231:dynamicdata)  [unwired: 3 in]
      n317 = call "Convert to Dynamic Data11"("Array"=w1216) -> ("Dynamic Data Type"=w1223:dynamicdata)  [unwired: 3 in]
      n318 = call "Convert to Dynamic Data13"("Array"=w1214) -> ("Dynamic Data Type"=w1219:dynamicdata)  [unwired: 3 in]
      n319 = call "Convert to Dynamic Data"("Array"=w1242) -> ("Dynamic Data Type"=w1241:dynamicdata)  [unwired: 3 in]
      n320 = call "Convert to Dynamic Data12"("Array"=w1215) -> ("Dynamic Data Type"=w1221:dynamicdata)  [unwired: 3 in]
      n321 = call "Convert to Dynamic Data10"("Array"=w1217) -> ("Dynamic Data Type"=w1225:dynamicdata)  [unwired: 3 in]
      n322 = call "Convert to Dynamic Data17"("Array"=w1200) -> ("Dynamic Data Type"=w1205:dynamicdata)  [unwired: 3 in]
      n323 = call "Convert to Dynamic Data18"("Array"=w1199) -> ("Dynamic Data Type"=w1203:dynamicdata)  [unwired: 3 in]
      n324 = call "Convert to Dynamic Data16"("Array"=w1201) -> ("Dynamic Data Type"=w1207:dynamicdata)  [unwired: 3 in]
      n325 = call "Convert to Dynamic Data15"("Array"=w1202) -> ("Dynamic Data Type"=w1209:dynamicdata)  [unwired: 3 in]
      n326 = call "Convert to Dynamic Data14"("Array"=w1212) -> ("Dynamic Data Type"=w1211:dynamicdata)  [unwired: 3 in]
      n327 = call "Convert to Dynamic Data2"("Array"=w1243) -> ("Dynamic Data Type"=w1240:dynamicdata)  [unwired: 3 in]
      n328 = call "Convert to Dynamic Data6"("Array"=w1229) -> ("Dynamic Data Type"=w1237:dynamicdata)  [unwired: 3 in]
      n329 = call "Convert to Dynamic Data8"("Array"=w1227) -> ("Dynamic Data Type"=w1233:dynamicdata)  [unwired: 3 in]
      n330 = call "Convert to Dynamic Data7"("Array"=w1228) -> ("Dynamic Data Type"=w1235:dynamicdata)  [unwired: 3 in]
      n331 = xnode "Set Dynamic Data Attributes"("Signals In"=w1240, "Signal Name"="Servo 1 Commanded Position") -> ("Signals Out"=w1198:dynamicdata)  [unwired: 2 in, 1 out]
      n332 = xnode "Set Dynamic Data Attributes"("Signals In"=w1237, "Signal Name"="Servo 2 Commanded Position") -> ("Signals Out"=w1197:dynamicdata)  [unwired: 2 in, 1 out]
      n333 = xnode "Set Dynamic Data Attributes"("Signals In"=w1233, "Signal Name"="Servo 4 Commanded Position") -> ("Signals Out"=w1195:dynamicdata)  [unwired: 2 in, 1 out]
      n334 = xnode "Set Dynamic Data Attributes"("Signals In"=w1235, "Signal Name"="Servo 3 Commanded Position") -> ("Signals Out"=w1196:dynamicdata)  [unwired: 2 in, 1 out]
      n335 = xnode "Set Dynamic Data Attributes"("Signals In"=w1231, "Signal Name"="Servo 5 Commanded Position") -> ("Signals Out"=w1194:dynamicdata)  [unwired: 2 in, 1 out]
      n336 = xnode "Set Dynamic Data Attributes"("Signals In"=w1241, "Signal Name"="Servo 1 Feedback Position") -> ("Signals Out"=w1193:dynamicdata)  [unwired: 2 in, 1 out]
      n337 = xnode "Set Dynamic Data Attributes"("Signals In"=w1221, "Signal Name"="Servo 1 Feedback Position") -> ("Signals Out"=w1190:dynamicdata)  [unwired: 2 in, 1 out]
      n338 = xnode "Set Dynamic Data Attributes"("Signals In"=w1223, "Signal Name"="Servo 1 Feedback Position") -> ("Signals Out"=w1191:dynamicdata)  [unwired: 2 in, 1 out]
      n339 = xnode "Set Dynamic Data Attributes"("Signals In"=w1205, "Signal Name"="Servo 4  Torque") -> ("Signals Out"=w1185:dynamicdata)  [unwired: 2 in, 1 out]
      n340 = xnode "Set Dynamic Data Attributes"("Signals In"=w1203, "Signal Name"="Servo 5  Torque") -> ("Signals Out"=w1184:dynamicdata)  [unwired: 2 in, 1 out]
      n341 = xnode "Set Dynamic Data Attributes"("Signals In"=w1225, "Signal Name"="Servo 1 Feedback Position") -> ("Signals Out"=w1192:dynamicdata)  [unwired: 2 in, 1 out]
      n342 = xnode "Set Dynamic Data Attributes"("Signals In"=w1207, "Signal Name"="Servo 3  Torque") -> ("Signals Out"=w1186:dynamicdata)  [unwired: 2 in, 1 out]
      n343 = xnode "Set Dynamic Data Attributes"("Signals In"=w1219, "Signal Name"="Servo 1 Feedback Position") -> ("Signals Out"=w1189:dynamicdata)  [unwired: 2 in, 1 out]
      n344 = xnode "Set Dynamic Data Attributes"("Signals In"=w1209, "Signal Name"="Servo 2  Torque") -> ("Signals Out"=w1187:dynamicdata)  [unwired: 2 in, 1 out]
      n345 = xnode "Set Dynamic Data Attributes"("Signals In"=w1211, "Signal Name"="Servo 1  Torque") -> ("Signals Out"=w1188:dynamicdata)  [unwired: 2 in, 1 out]
      n346 = Merge Signals(w1198, w1197, w1196, w1195, w1194, w1193, w1192, w1191, w1190, w1189, w1188, w1187, w1186, w1185, w1184) -> (w1183:dynamicdata)
      n347 = call "Write To Measurement File"("Signals"=w1183, "Filename"="Filename", "Comment"="Comment") -> ()  [unwired: 14 in, 3 out]
    }
  }
